vi "FSPL_CALC.vi"(1 "f":dbl format="%#_13g", 3 "d":dbl format="%#_13g", 5 "error in":errorcluster, 8 "Ant1 Gain (dB)":dbl format="%#_13g", 9 "f(units)":u16(ring) items=["GHz", "MHz"], 10 "Ant2 Gain dB":dbl format="%#_13g", 11 "d(units)":u16(ring)=2 items=["Meter", "Feet", "Inches"]) -> (15 "Corr(dB)":dbl, 17 "fsl(dB)":dbl, 19 "error out":errorcluster)   [LabVIEW 2018]
panel:
  out "# of W":dbl
  out "Wavelength":dbl
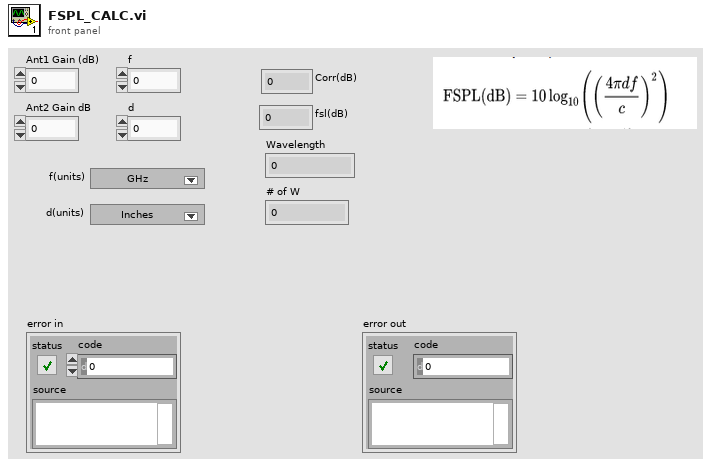
[diagram p1: front panel]
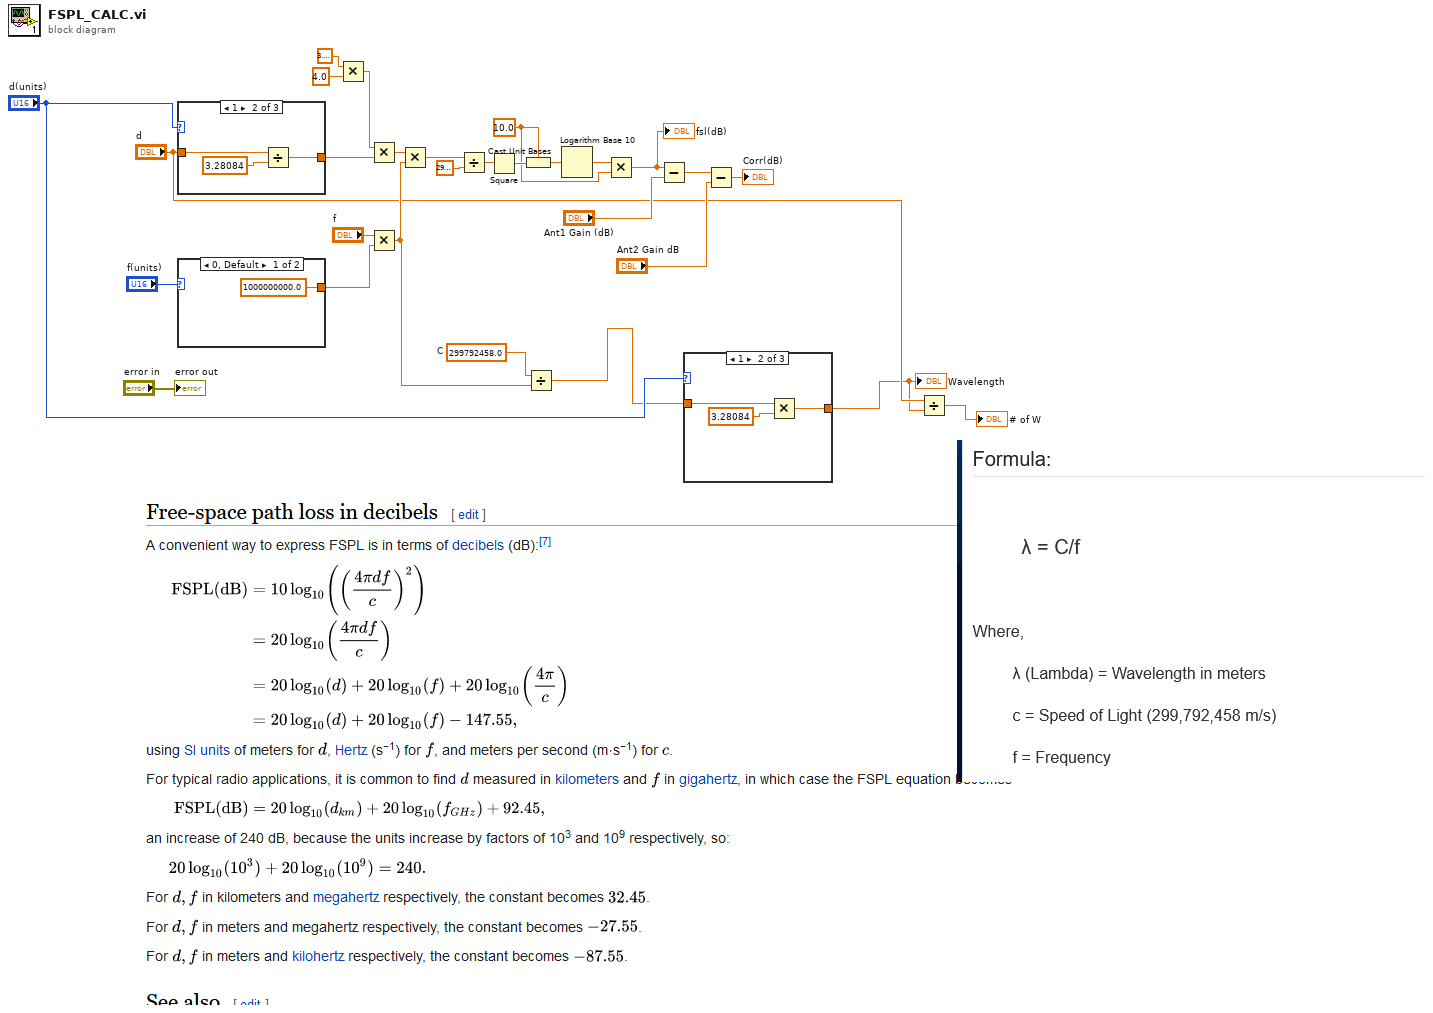
[diagram p0: block diagram]
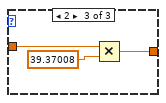
[diagram p3: hidden frame]
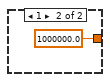
[diagram p4: hidden frame]
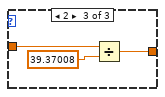
[diagram p6: hidden frame]
diagram:
  w8 = 299792458.0  # C
  w16 = 10.0 ("unit (none)")
  n1 = case shown="1" "d(units)" {
    tunnel: "d" -> [w29 w32 w35]
    tunnel: [w29 w30 w33] -> w4
    frame 0, Default {
    }
    frame 1 {
      n2 = Divide(x=w32, y=3.28084) -> (x/y=w30:dbl)
    }
    frame 2 {
      n3 = Divide(x=w35, y=39.37008) -> (x/y=w33:dbl)
    }
  }
  n4 = case shown="0, Default" "f(units)" {
    tunnel: [1000000000.0 ("y") 1000000.0 ("y")] -> w21
    frame 0, Default {
    }
    frame 1 {
    }
  }
  n5 = Multiply(x=3.141592653589793, y=4.0) -> (x*y=w26:dbl)
  n6 = Multiply(x=w26, y=w4) -> (x*y=w25:dbl)
  n7 = Multiply(x="f", y=w21) -> (x*y=w7:dbl)
  n8 = Multiply(x=w25, y=w7) -> (x*y=w23:dbl)
  n9 = Divide(x=w23, y=dbl[unit] 299792458.0) -> (x/y=w20:dbl[unit])
  n10 = Square(x=w20) -> (x^2=w17:dbl[unit])
  n11 = Cast Unit Bases(0:w17, 1:w16) -> (2:w18:dbl)
  n12 = Divide(x=w8, y=w7) -> (x/y=w5:dbl)
  n13 = Logarithm Base 10(1:w18) -> (0:w19:dbl)
  n14 = Multiply(x=w19, y=w16) -> (x*y=w13:dbl)
  "fsl(dB)" <- w13
  n15 = Subtract(x=w13, y="Ant1 Gain (dB)") -> (x-y=w11:dbl)
  n16 = case shown="1" "d(units)" {
    tunnel: w5 -> [w38 w41 w44]
    tunnel: [w38 w39 w42] -> w1
    frame 0, Default {
    }
    frame 1 {
      n17 = Multiply(x=w41, y=3.28084) -> (x*y=w39:dbl)
    }
    frame 2 {
      n18 = Multiply(x=w44, y=39.37008) -> (x*y=w42:dbl)
    }
  }
  "Wavelength" <- w1
  n19 = Subtract(x=w11, y="Ant2 Gain dB") -> (x-y=→"Corr(dB)":dbl)
  n20 = Divide(x="d", y=w1) -> (x/y=→"# of W":dbl)
  "error out" <- "error in"
